vi "Replace_Shortcut.vi"(8 "error in (no error)":errorcluster, 9 "shortcut address":string, 10 "shortcut":refnum<class "IB_Shortcut.lvclass">, 11 "IB_Source_File in":refnum<class "IB_Source_File.lvclass">) -> (0 "error out":errorcluster, 3 "IB_Source_File out":refnum<class "IB_Source_File.lvclass">)   [LabVIEW 2020, in "IB_Source_File.lvclass"]
uses:
  <vilib>/AppBuilder/IB_Classes/Source/File/IB_Source_File.lvclass
  <vilib>/AppBuilder/IB_Classes/Source/File/IB_Source_File.lvclass/IB_Source_File.ctl
  <vilib>/AppBuilder/IB_Classes/Shortcut/IB_Shortcut.lvclass
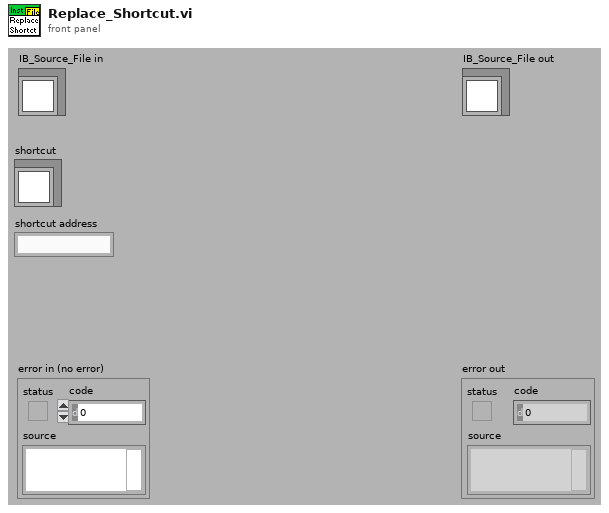
[diagram p1: front panel]
types:
  T1 = typedef "IB_Source_File.ctl" = cluster{"Attributes":i16, "RegCOM":bool, "unlock":bool, "shortcuts":refnum<class "IB_Shortcut.lvclass">[], "EXE_install":bool, "CmdArg_install":string, "EXE_uninstall":bool, "CmdArg_uninstall":string}
  T2 = typedef "IB_Shortcut.ctl" = cluster{"name":string, "destIndex":i32, "subDir":string, "address":string}
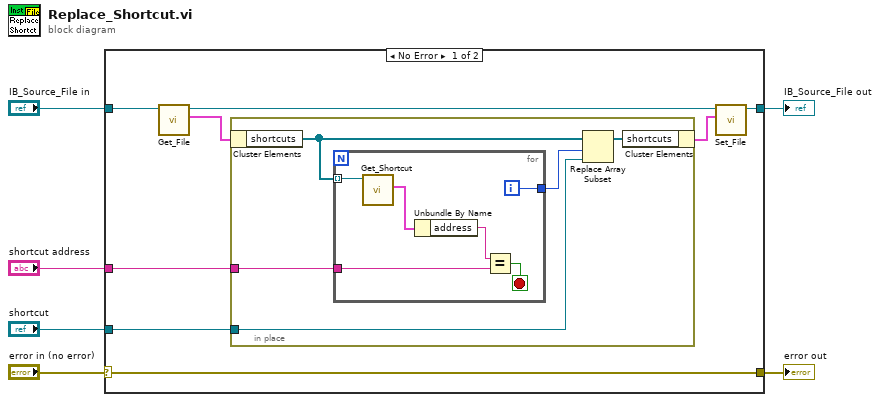
[diagram p0: block diagram]
diagram:
  n1 = case shown="No Error" "error in (no error)" {
    selector: "error in (no error)" -> [w14 w27]
    tunnel: [w14 w27] -> w5
    tunnel: [w9 w26] -> w3
    tunnel: "IB_Source_File in" -> [w10 w26]
    tunnel: "shortcut address" -> [w8 _]
    tunnel: "shortcut" -> [w7 _]
    frame No Error {
      n2 = call <vilib>:"Get_File.vi"("IB_Source_File in"=w10) -> ("data"=w12:T1, "IB_Source_File out"=w13:refnum<class "IB_Source_File.lvclass">)  [unwired: 1 in, 8 out]
      n3 = in-place {
        in-place-border: w8 -> [w19]
        in-place-border: w7 -> [w17]
        n4 = in-place-cluster #1(w12) -> ("shortcuts"=w16:refnum<class "IB_Shortcut.lvclass">[])
        n5 = for {
          tunnel: w16 -> [w25] mode=indexing
          tunnel: w19 -> [w23]
          tunnel: [w21] -> w18
          i -> [w21]
          stop <- w22 stop-if-true
          n6 = call <vilib>:"Get_Shortcut.vi"("Class in"=w25) -> ("data"=w24:T2)  [unwired: 1 in, 9 out]
          n7 = Unbundle By Name(w24) -> ("address"=w20:string)
          n8 = Equal?(x=w20, y=w23) -> (x = y?=w22:bool)
        }
        n9 = Replace Array Subset(array=w16, new element=w17, index=w18) -> (w15:refnum<class "IB_Shortcut.lvclass">[])
        n10 = in-place-cluster #1("shortcuts"=w15) -> (w11:T1)
      }
      n11 = call <vilib>:"Set_File.vi"("data"=w11, "IB_Source_File in"=w13) -> ("IB_Source_File out"=w9:refnum<class "IB_Source_File.lvclass">)  [unwired: 1 in, 8 out]
    }
    frame Error {
    }
  }
  "error out" <- w5
  "IB_Source_File out" <- w3
